vi "fit function - sine.vi"(3 "output control":T1, 4 "data":T2, 5 "X":dbl[](array[numeric]), 6 "a":dbl[](array[numeric])) -> (0 "error out":errorcluster, 1 "f'(X,a)":dbl[][](array[numeric]), 2 "f(X,a)":dbl[](array[numeric]))   [LabVIEW 2012]
doc: "This template is the starting point for creating a model function to be passed to the Nonlinear Curve Fit.vi."
uses:
  <vilib>/gmath/NumericalOptimization/objective function data.ctl
  <vilib>/gmath/NumericalOptimization/LM_output select.ctl
  <vilib>/gmath/NI_Gmath.lvlib
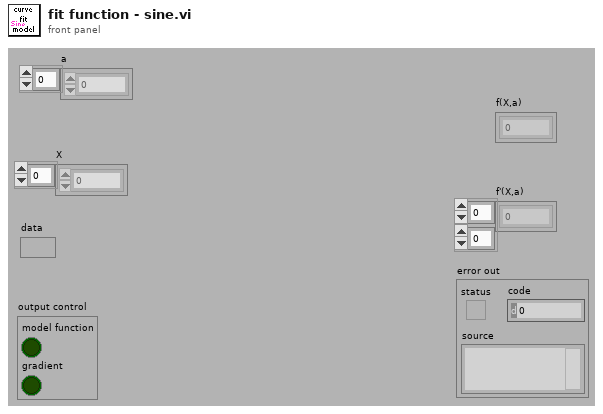
[diagram p1: front panel]
types:
  T1 = typedef "NI_Gmath.lvlib/LM_output select.ctl" = cluster{"model function":bool, "gradient":bool}
  T2 = typedef "NI_Gmath.lvlib/objective function data.ctl" = variant
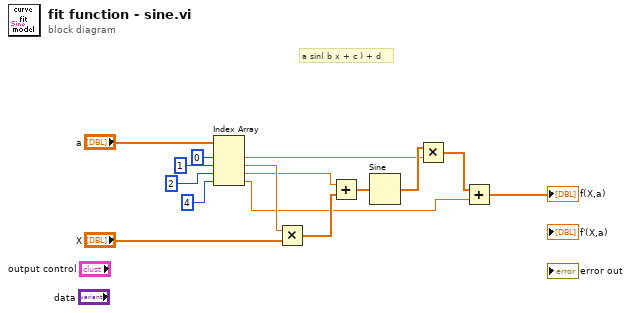
[diagram p0: block diagram]
diagram:
  # "a sin( b x + c ) + d"
  n1 = Index Array(array="a", index #1=0 ("index"), index #2=1 ("index"), index #3=2 ("index"), index #4=4 ("index")) -> (element #1=w3:dbl, element #2=w8:dbl, element #3=w6:dbl, element #4=w1:dbl)
  n2 = Multiply(x=w8, y="X") -> (x*y=w7:dbl[])
  n3 = Add(x=w6, y=w7) -> (x+y=w5:dbl[])
  n4 = Sine(x=w5) -> (sin(x)=w4:dbl[])
  n5 = Multiply(x=w4, y=w3) -> (x*y=w2:dbl[])
  n6 = Add(x=w2, y=w1) -> (x+y=→"f(X,a)":dbl[])
